vi "unflattenPlaneAngleFromXML_Array.vi"(8 "error in (no error)":errorcluster, 9 "planeAngleUnitInXML":T1, 10 "xmlString":string, 11 "planeAngleForType":dbl[unit][](array[numeric])=[0.004569261296800628, 0.009138522593601256, 0.013707783890401884, 0.018277045187202513]) -> (0 "error out":errorcluster, 3 "planeAngle":dbl[unit][](array[numeric]))   [LabVIEW 2016, in "UnitsAndXML.lvlib"]
uses:
  <userlib>/Common/UnitsAndXML/UnitsAndXML.lvlib
  <userlib>/Common/UnitsAndXML/FlattenItemWithUnitToXML/FlattenPlaneAngleToXML/PlaneAngleUnit.ctl
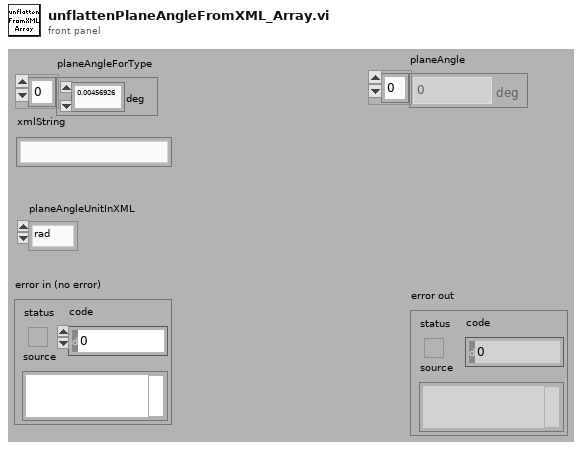
[diagram p1: front panel]
types:
  T1 = typedef "UnitsAndXML.lvlib/PlaneAngleUnit.ctl" = enum16{"rad", "deg", "'", "\""}
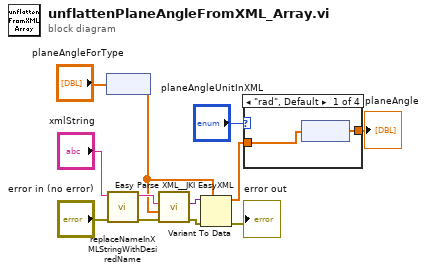
[diagram p0: block diagram]
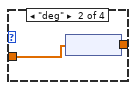
[diagram p2: hidden frame]
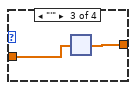
[diagram p3: hidden frame]
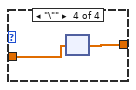
[diagram p4: hidden frame]
diagram:
  n1 = node("planeAngleForType") -> (w8:dbl[])
  n2 = call <userlib>:"replaceNameInXMLStringWithDesiredName.vi"("error in"="error in (no error)", "xmlString"="xmlString") -> ("error out"=w1:errorcluster, "revisedXMLString"=w9:string)  [unwired: 8 in]
  n3 = call <vilib>:"Easy Parse XML__JKI EasyXML.vi"("error in (no error)"=w1, "LabVIEW Data (Type)"=w8, "XML String"=w9) -> ("error out"=w4:errorcluster, "LabVIEW Data"=w11:variant)  [unwired: 7 in]
  n4 = Variant To Data(error in=w4, type=w8, Variant=w11) -> (data=w7:dbl[], error out=→"error out":errorcluster)
  n5 = case shown="\"rad\", Default" "planeAngleUnitInXML" {
    tunnel: w7 -> [w13 w16 w18 w20]
    tunnel: [w14 w15 w17 w19] -> w6
    frame "rad", Default {
      n6 = node(w13) -> (w14:dbl[unit][])
    }
    frame "deg" {
      n7 = node(w16) -> (w15:dbl[unit][])
    }
    frame "'" {
      n8 = node(w18) -> (w17:dbl[unit][])
    }
    frame "\"" {
      n9 = node(w20) -> (w19:dbl[unit][])
    }
  }
  "planeAngle" <- w6
